vi "Shutdown.vi"(8 "error in":errorcluster, 9 "timeout in ms (-1)":i32=-1, 11 "LVTM_Plugin":refnum<class "LVTM_Plugin.lvclass">) -> (0 "error out":errorcluster, 3 "LVTM_Plugin Out":refnum<class "LVTM_Plugin.lvclass">)   [LabVIEW 2013, in "LVTM_Plugin.lvclass"]
uses:
  LVTM_Plugin.lvclass
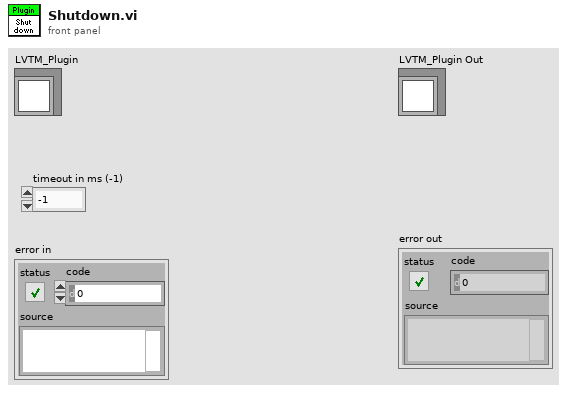
[diagram p1: front panel]
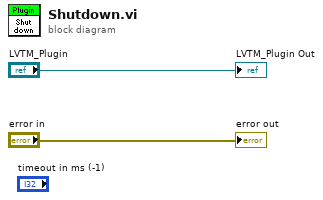
[diagram p0: block diagram]
diagram:
  "LVTM_Plugin Out" <- "LVTM_Plugin"
  "error out" <- "error in"
